vi "XOR5.vi"(11 "inputs":T1={"Button 1"=TRUE, "Button 2"=TRUE, "Button 3"=TRUE, "Button 4"=TRUE, "Button 5"=FALSE}) -> (3 "XOR5":bool)   [LabVIEW 2015]
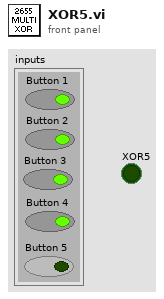
[diagram p1: front panel]
types:
  T1 = cluster{"Button 1":bool, "Button 2":bool, "Button 3":bool, "Button 4":bool, "Button 5":bool}
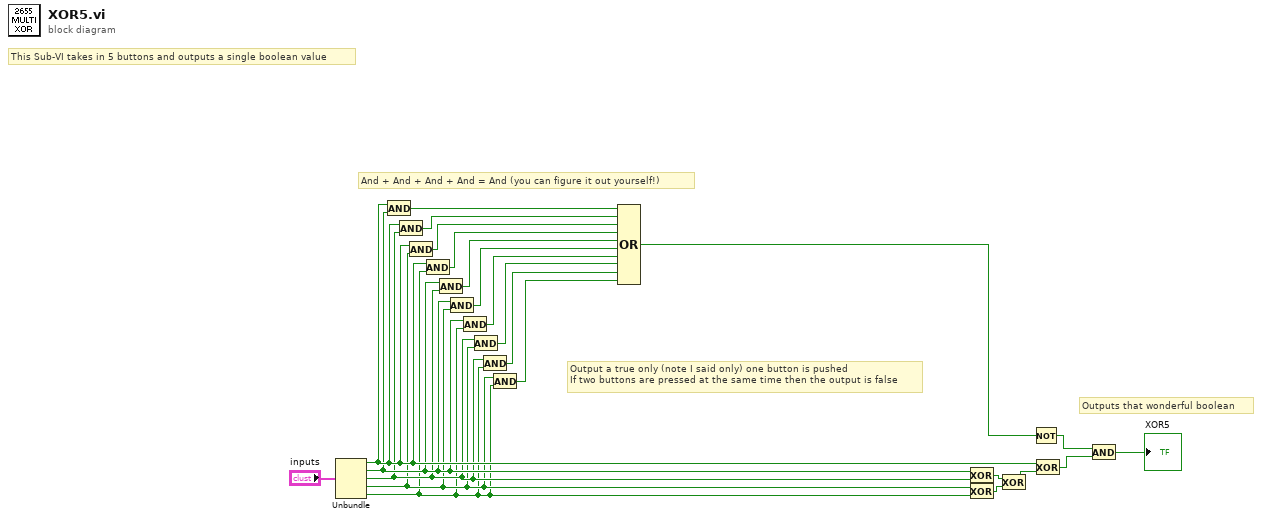
[diagram p0: block diagram]
diagram:
  # "Output a true only (note I said only) one button is pushed\nIf two buttons are pressed at the same time then the output is false"
  # "Outputs that wonderful boolean"
  # "And + And + And + And = And (you can figure it out yourself!)"
  # "This Sub-VI takes in 5 buttons and outputs a single boolean value"
  n1 = Unbundle("inputs") -> ("Button 1"=w19:bool, "Button 2"=w18:bool, "Button 3"=w17:bool, "Button 4"=w16:bool, "Button 5"=w15:bool)
  n2 = And(x=w19, y=w18) -> (x .and. y?=w14:bool)
  n3 = And(x=w19, y=w17) -> (x .and. y?=w13:bool)
  n4 = And(x=w19, y=w16) -> (x .and. y?=w12:bool)
  n5 = And(x=w19, y=w15) -> (x .and. y?=w11:bool)
  n6 = And(x=w18, y=w17) -> (x .and. y?=w10:bool)
  n7 = And(x=w18, y=w16) -> (x .and. y?=w9:bool)
  n8 = And(x=w18, y=w15) -> (x .and. y?=w8:bool)
  n9 = And(x=w17, y=w16) -> (x .and. y?=w7:bool)
  n10 = And(x=w17, y=w15) -> (x .and. y?=w6:bool)
  n11 = And(x=w16, y=w15) -> (x .and. y?=w5:bool)
  n12 = Compound Arithmetic op=OR(w14, w13, w12, w11, w10, w9, w8, w7, w6, w5) -> (w4:bool)
  n13 = Exclusive Or(1:w17, 2:w18) -> (0:w23:bool)
  n14 = Exclusive Or(1:w15, 2:w16) -> (0:w22:bool)
  n15 = Exclusive Or(1:w22, 2:w23) -> (0:w21:bool)
  n16 = Not(x=w4) -> (.not. x?=w3:bool)
  n17 = Exclusive Or(1:w21, 2:w19) -> (0:w2:bool)
  n18 = And(x=w3, y=w2) -> (x .and. y?=→"XOR5":bool)
